vi "Create chrip signal.vi"(4 "type":u16(ring) items=["Linear", "Logarithmic"], 6 "Fs":sgl=3072000000.0 format="%#_6p", 9 "F 2":sgl, 10 "F 1":sgl, 11 "Samples":i32) -> (1 "dt":sgl, 2 "I16":i16[](array[numeric]), 3 "SGL":csg[](array[numeric]))   [LabVIEW 2019]
uses:
  <vilib>/Analysis/1siggen.llb/Ramp Pattern by Samples.vi
  <vilib>/Analysis/NI_AALBase.lvlib
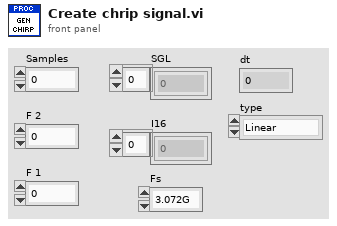
[diagram p1: front panel]
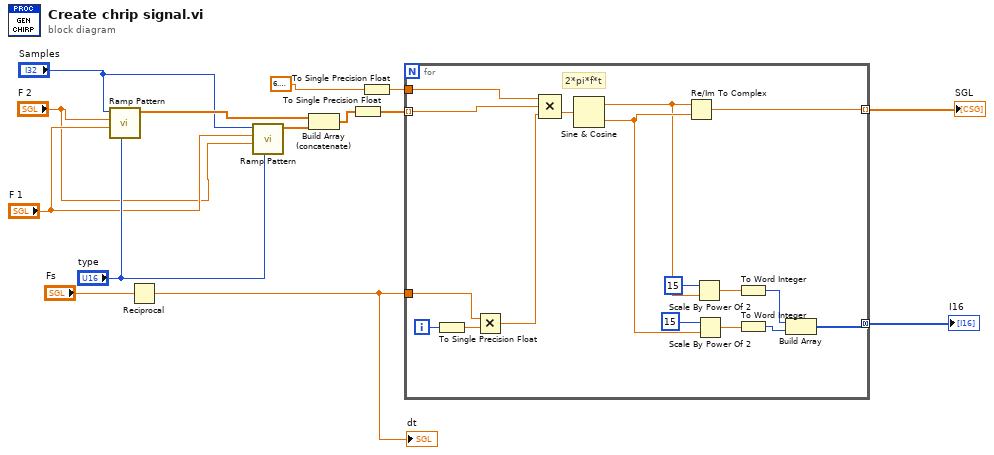
[diagram p0: block diagram]
diagram:
  n1 = call-poly <vilib>:"Ramp Pattern.vi"("type"="type", "start"="F 1", "end"="F 2", "samples"="Samples") -> ("Ramp Pattern"=w8:dbl[])  [unwired: 6 in, 1 out]
  n2 = Reciprocal(x="Fs") -> (1/x=w12:sgl)
  "dt" <- w12
  n3 = call-poly <vilib>:"Ramp Pattern.vi"("type"="type", "start"="F 2", "end"="F 1", "samples"="Samples") -> ("Ramp Pattern"=w1:dbl[])  [unwired: 6 in, 1 out]
  n4 = Build Array (concatenate)(w8, w1) -> (w2:dbl[])
  n5 = To Single Precision Float(number=w2) -> (single precision float=w9:sgl[])
  n6 = To Single Precision Float(number=6.283185307179586) -> (single precision float=w11:sgl)
  n7 = for {
    tunnel: w12 -> [w29]
    tunnel: w9 -> [w28] mode=indexing
    tunnel: w11 -> [w27]
    tunnel: [w24] -> w14 mode=indexing
    tunnel: [w16] -> w13 mode=concatenating
    i -> [w31]
    # "2*pi*f*t"
    n8 = To Single Precision Float(number=w31) -> (single precision float=w30:sgl)
    n9 = Multiply(x=w29, y=w30) -> (x*y=w26:sgl)
    n10 = Compound Arithmetic op=MULTIPLY(w27, w28, w26) -> (w25:sgl)
    n11 = Sine & Cosine(0:w25) -> (1:w15:sgl, 2:w23:sgl)
    n12 = Re/Im To Complex(1:w23, 2:w15) -> (0:w24:csg)
    n13 = Scale By Power Of 2(n=i16 15, x=w15) -> (x*2^n=w20:sgl)
    n14 = Scale By Power Of 2(n=i16 15, x=w23) -> (x*2^n=w19:sgl)
    n15 = To Word Integer(number=w20) -> (16bit integer=w17:i16)
    n16 = To Word Integer(number=w19) -> (16bit integer=w18:i16)
    n17 = Build Array(w17, w18) -> (w16:i16[])
  }
  "SGL" <- w14
  "I16" <- w13
